vi "Find T0 and dTt.vi"(7 "Check Option":T1(ring), 11 "Array":dbl[](array[numeric])) -> (1 "dT":dbl, 3 "T0":dbl)   [LabVIEW 2020, in "TEXT.lvclass"]
uses:
  TEXT.lvclass
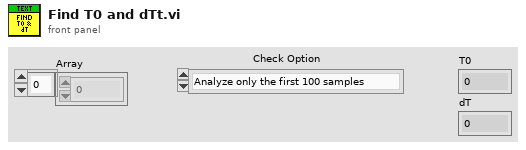
[diagram p1: front panel]
types:
  T1 = enum16{"Analyze only the first 100 samples", "Analyze the complete signal"}
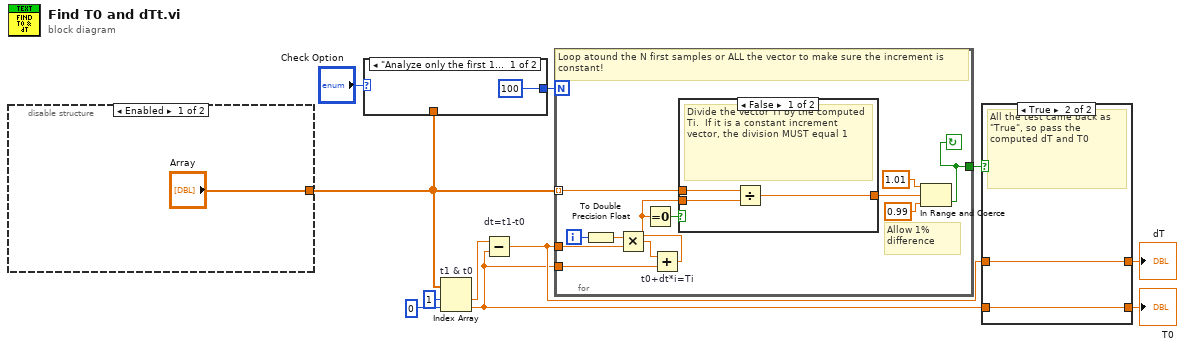
[diagram p0: block diagram]
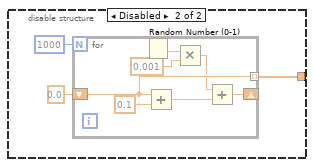
[diagram p2: hidden frame]
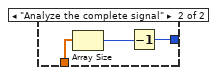
[diagram p3: hidden frame]
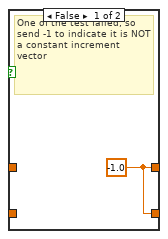
[diagram p4: hidden frame]
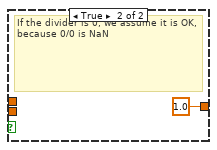
[diagram p5: hidden frame]
diagram:
  n1 = disable-structure shown="Enabled" {
    disable-tunnel: ["Array" w14] -> w6
    frame Enabled {
    }
    frame Disabled {
      n2 = for {
        N: 1000 -> [_]
        shift-right: [w19] -> _
        shift-left: 0.0 -> [w20]
        tunnel: [w20] -> w14 mode=indexing
        n3 = Random Number (0-1)() -> (number: 0 to 1=w18:dbl)
        n4 = Add(x=w20, y=0.1) -> (x+y=w22:dbl)
        n5 = Multiply(x=w18, y=0.001) -> (x*y=w17:dbl)
        n6 = Add(x=w17, y=w22) -> (x+y=w19:dbl)
      }
    }
  }
  n7 = case shown="\"Analyze only the first 100 samples\", Default" "Check Option" {
    tunnel: [100 w24] -> w7
    tunnel: w6 -> [_ w25]
    frame "Analyze only the first 100 samples", Default {
    }
    frame "Analyze the complete signal" {
      n8 = Array Size(array=w25) -> (size(s)=w26:i32)
      n9 = Decrement(x=w26) -> (x-1=w24:i32)
    }
  }
  n10 = Index Array "t1 & t0"(array=w6, index #1=1 ("index"), index #2=0 ("index")) -> (element #1=w4:dbl, element #2=w2:dbl)
  n11 = Subtract "dt=t1-t0"(x=w4, y=w2) -> (x-y=w3:dbl)
  n12 = for {
    N: w7 -> [_]
    tunnel: w3 -> [w38]
    tunnel: w2 -> [w35]
    tunnel: w6 -> [w27] mode=indexing
    tunnel: [w28] -> w1
    i -> [w30]
    stop <- w28 continue-if-true
    # "Allow 1% difference"
    # "Loop atound the N first samples or ALL the vector to make sure the increment is constant!"
    n13 = To Double Precision Float(number=w30) -> (double precision float=w37:dbl)
    n14 = Multiply(x=w37, y=w38) -> (x*y=w36:dbl)
    n15 = Add "t0+dt*i=Ti"(x=w36, y=w35) -> (x+y=w29:dbl)
    n16 = Equal To 0?(x=w29) -> (x = 0?=w31:bool)
    n17 = case shown="False" w31 {
      tunnel: w29 -> [w41 _]
      tunnel: [w40 1.0] -> w34
      tunnel: w27 -> [w39 _]
      frame False {
        # "Divide the vector Ti by the computed Ti.  If it is a constant increment vector, the division MUST equal 1"
        n18 = Divide(x=w39, y=w41) -> (x/y=w40:dbl)
      }
      frame True {
        # "If the divider is 0, we assume it is OK, because 0/0 is NaN"
      }
    }
    n19 = In Range and Coerce(upper limit=1.01 ("lower limit"), x=w34, lower limit=0.99 ("upper limit")) -> (In Range?=w28:bool)  [unwired: 1 out]
  }
  n20 = case shown="True" w1 {
    tunnel: [w43 w45] -> w10
    tunnel: w2 -> [_ w45]
    tunnel: [w43 w44] -> w9
    tunnel: w3 -> [_ w44]
    frame False {
      w43 = -1.0
      # "One of the test failed, so send -1 to indicate it is NOT a constant increment vector"
    }
    frame True {
      # "All the test came back as \"True\", so pass the computed dT and T0"
    }
  }
  "T0" <- w10
  "dT" <- w9
